vi "getTableCount.vi"(8 "error in (no error)":errorcluster, 11 ".NET Refnum in":refnum<k24>) -> (0 "error out":errorcluster, 2 "Table Count":i32, 3 ".NET Refnum out":refnum<k24>)   [LabVIEW 2017, in "LabVIEW NPOI.lvlib" / "xwpfReader.lvclass"]
uses:
  xwpfReader.lvclass
  C:/Users/Neo/Desktop/Dev_Tools_BR/LabVIEW_NPOI/lib/NPOI 2.1.1/NPOI.OOXML.dll
  lib/NPOI 2.1.1/NPOI.OOXML.dll
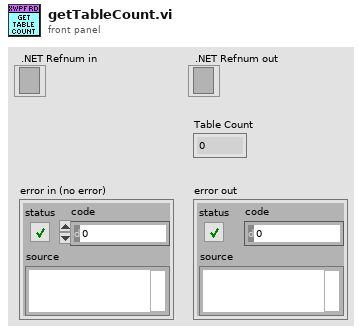
[diagram p1: front panel]
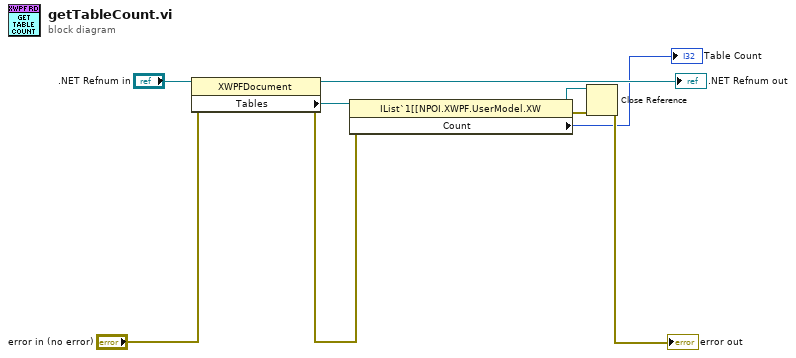
[diagram p0: block diagram]
diagram:
  n1 = property class="XWPFDocument"(reference=".NET Refnum in", error in="error in (no error)") -> (reference out=→".NET Refnum out":refnum<k24>, error out=w5:errorcluster, "Tables"=w2:refnum<k24>)
  n2 = property class="IList`1[[NPOI.XWPF.UserModel.XW"(reference=w2, error in=w5) -> (reference out=w7:refnum<k24>, error out=w8:errorcluster, "Count"=→"Table Count":i32)
  n3 = Close Reference(reference=w7, error in (no error)=w8) -> (error out=→"error out":errorcluster)
